vi "Software Commands.vi"() -> ()   [LabVIEW 2015]
panel:
  in  "Aalborg DFC Software Interface Commands":T1(array[cluster])=[{"Command Name"="Mode", "Description"="sets analog mode", "Number"="1", "Command"="M", "Argument 1"="A", "Argument 2"="", "Argument 3"="", "Argument 4"="", "Response"="MA"}, {"Command Name"="Mode", "Description"="set digital mode", "Number"="1", "Command"="M", "Argument 1"="D", "Argument 2"="", "Argument 3"="", "Argument 4"="", "Response"="MD"}, {"Command Name"="Mode", "Description"="returns status", "Number"="1", "Command"="M", "Argument 1"="S", "Argument 2"="", "Argument 3"="", "Argument 4"="", "Response"="MA or MD"}, {"Command Name"="Set Point", "Description"="send desired flow setting (digital mode)", "Number"="2", "Command"="S", "Argument 1"="<Value>", "Argument 2"="", "Argument 3"="", "Argument 4"="", "Response"="S <Value>"}, {"Command Name"="Flow", "Description"="request sensor reading", "Number"="3", "Command"="F", "Argument 1"="", "Argument 2"="", "Argument 3"="", "Argument 4"="", "Response"="<Value>"}, {"Command Name"="Valve", "Description"="R/W op mode of ctl valve - Auto", "Number"="4", "Command"="V", "Argument 1"="A", "Argument 2"="", "Argument 3"="", "Argument 4"="", "Response"="VA"}, {"Command Name"="Valve", "Description"="R/W op mode of ctl valve - Force Open", "Number"="4", "Command"="V", "Argument 1"="O", "Argument 2"="", "Argument 3"="", "Argument 4"="", "Response"="VO"}, {"Command Name"="Valve", "Description"="R/W op mode of ctl valve - Force Closed", "Number"="4", "Command"="V", "Argument 1"="C", "Argument 2"="", "Argument 3"="", "Argument 4"="", "Response"="VC"}, {"Command Name"="Valve", "Description"="R/W op mode of ctl valve - Return Status", "Number"="4", "Command"="V", "Argument 1"="S", "Argument 2"="", "Argument 3"="", "Argument 4"="", "Response"="VA, VO or VC"}, {"Command Name"="Gas Select", "Description"="sel 1/10 gas cals", "Number"="5", "Command"="G", "Argument 1"="<0:1:9>", "Argument 2"="", "Argument 3"="", "Argument 4"="", "Response"="G1 thru G10"}, {"Command Name"="Auto Zero", "Description"="R/W auto zero - enable, do when SP<2%FS", "Number"="6", "Command"="Z", "Argument 1"="E", "Argument 2"="", "Argument 3"="", "Argument 4"="", "Response"="ZE"}, {"Command Name"="Auto Zero", "Description"="R/W auto zero - disable", "Number"="6", "Command"="Z", "Argument 1"="D", "Argument 2"="", "Argument 3"="", "Argument 4"="", "Response"="ZD"}, {"Command Name"="Auto Zero", "Description"="R/W auto zero - do it now", "Number"="6", "Command"="Z", "Argument 1"="N", "Argument 2"="", "Argument 3"="", "Argument 4"="", "Response"="ZN"}, {"Command Name"="Auto Zero", "Description"="R/W auto zero - write zero to SDPROC", "Number"="6", "Command"="Z", "Argument 1"="W", "Argument 2"="", "Argument 3"="", "Argument 4"="", "Response"="ZW"}, {"Command Name"="Auto Zero", "Description"="R/W auto zero - status", "Number"="6", "Command"="Z", "Argument 1"="S", "Argument 2"="", "Argument 3"="", "Argument 4"="", "Response"="ZE, ZD, or ZIN <value>"}, {"Command Name"="Flow Alarms", "Description"="R/W status of gas flow alarms - high dev", "Number"="7", "Command"="A", "Argument 1"="<Value>", "Argument 2"="", "Argument 3"="", "Argument 4"="", "Response"="AH"}, {"Command Name"="Flow Alarms", "Description"="R/W status of gas flow alarms - low dev", "Number"="7", "Command"="A", "Argument 1"="<Value>", "Argument 2"="", "Argument 3"="", "Argument 4"="", "Response"="AL"}, {"Command Name"="Flow Alarms", "Description"="R/W status of gas flow alarms - disable", "Number"="7", "Command"="A", "Argument 1"="", "Argument 2"="", "Argument 3"="", "Argument 4"="", "Response"="AD"}, {"Command Name"="Flow Alarms", "Description"="R/W status of gas flow alarms - status", "Number"="7", "Command"="A", "Argument 1"="", "Argument 2"="", "Argument 3"="", "Argument 4"="", "Response"="N, H, or L"}, {"Command Name"="Relay Action", "Description"="energize relay <Arg 1> when Arg 2 = true - disable", "Number"="8", "Command"="R", "Argument 1"="<1,2>", "Argument 2"="N", "Argument 3"="", "Argument 4"="", "Response"="RN"}, {"Command Name"="Relay Action", "Description"="energize relay <Arg 1> when Arg 2 = true - totalizer > limit", "Number"="8", "Command"="R", "Argument 1"="<1,2>", "Argument 2"="T", "Argument 3"="", "Argument 4"="", "Response"="RT"}, {"Command Name"="Relay Action", "Description"="energize relay <Arg 1> when Arg 2 = true - hi alarm", "Number"="8", "Command"="R", "Argument 1"="<1,2>", "Argument 2"="H", "Argument 3"="", "Argument 4"="", "Response"="RH"}, {"Command Name"="Relay Action", "Description"="energize relay <Arg 1> when Arg 2 = true - lo alarm", "Number"="8", "Command"="R", "Argument 1"="<1,2>", "Argument 2"="L", "Argument 3"="", "Argument 4"="", "Response"="RL"}, {"Command Name"="Relay Action", "Description"="energize relay <Arg 1> when Arg 2 = true - lo < range < hi", "Number"="8", "Command"="R", "Argument 1"="<1,2>", "Argument 2"="R", "Argument 3"="", "Argument 4"="", "Response"="RR"}, {"Command Name"="Relay Action", "Description"="relay <Arg 1> - status", "Number"="8", "Command"="R", "Argument 1"="<1,2>", "Argument 2"="S", "Argument 3"="", "Argument 4"="", "Response"="RN, RT, RH, RL, RR"}, {"Command Name"="Totalizer", "Description"="ctl totalizer - zero", "Number"="9", "Command"="T", "Argument 1"="Z", "Argument 2"="", "Argument 3"="", "Argument 4"="", "Response"="TZ"}, {"Command Name"="Totalizer", "Description"="ctl totalizer - start", "Number"="9", "Command"="T", "Argument 1"="S", "Argument 2"="<N,F>", "Argument 3"="<Value>", "Argument 4"="", "Response"="TSN, TS <value>"}, {"Command Name"="Totalizer", "Description"="ctl totalizer - stop", "Number"="9", "Command"="T", "Argument 1"="P", "Argument 2"="<N,T>", "Argument 3"="<Value>", "Argument 4"="", "Response"="TPN, TPT {N/C} <valve>"}, {"Command Name"="Totalizer", "Description"="ctl totalizer - read", "Number"="9", "Command"="T", "Argument 1"="R", "Argument 2"="", "Argument 3"="", "Argument 4"="", "Response"="<value>"}, {"Command Name"="Totalizer", "Description"="ctl totalizer - disable", "Number"="9", "Command"="T", "Argument 1"="D", "Argument 2"="", "Argument 3"="", "Argument 4"="", "Response"="TD"}, {"Command Name"="K Factors", "Description"="gas correction factor - disable (K = 1)", "Number"="10", "Command"="K", "Argument 1"="D", "Argument 2"="", "Argument 3"="", "Argument 4"="", "Response"="KD"}, {"Command Name"="K Factors", "Description"="gas correction factor - internal table", "Number"="10", "Command"="K", "Argument 1"="I", "Argument 2"="<index>", "Argument 3"="", "Argument 4"="", "Response"="KI <index> <name> <value>"}, {"Command Name"="K Factors", "Description"="gas correction factor - user specified factor", "Number"="10", "Command"="K", "Argument 1"="E", "Argument 2"="<value>", "Argument 3"="", "Argument 4"="", "Response"="KE <value>"}, {"Command Name"="Units", "Description"="set units - %FS", "Number"="11", "Command"="U", "Argument 1"="%", "Argument 2"="", "Argument 3"="", "Argument 4"="", "Response"="U%"}, {"Command Name"="Units", "Description"="set units - SLPM", "Number"="11", "Command"="U", "Argument 1"="SLPM", "Argument 2"="", "Argument 3"="", "Argument 4"="", "Response"="USLPM"}, {"Command Name"="Units", "Description"="set units - SLPH", "Number"="11", "Command"="U", "Argument 1"="SLPH", "Argument 2"="", "Argument 3"="", "Argument 4"="", "Response"="USLPH"}, {"Command Name"="Units", "Description"="set units - MLPM", "Number"="11", "Command"="U", "Argument 1"="MLPM", "Argument 2"="", "Argument 3"="", "Argument 4"="", "Response"="UMLPM"}, {"Command Name"="Units", "Description"="set units - MLPH", "Number"="11", "Command"="U", "Argument 1"="MLPH", "Argument 2"="", "Argument 3"="", "Argument 4"="", "Response"="UMLPH"}, {"Command Name"="Units", "Description"="set units - SCFH", "Number"="11", "Command"="U", "Argument 1"="SCFH", "Argument 2"="", "Argument 3"="", "Argument 4"="", "Response"="USCFH"}, {"Command Name"="Units", "Description"="set units - SCFM", "Number"="11", "Command"="U", "Argument 1"="SCFM", "Argument 2"="", "Argument 3"="", "Argument 4"="", "Response"="USCFM"}, {"Command Name"="Units", "Description"="set units - LBPH", "Number"="11", "Command"="U", "Argument 1"="LBPH", "Argument 2"="", "Argument 3"="", "Argument 4"="", "Response"="ULBPH"}, {"Command Name"="Units", "Description"="set units - LBPM", "Number"="11", "Command"="U", "Argument 1"="LBPM", "Argument 2"="", "Argument 3"="", "Argument 4"="", "Response"="ULBPM"}, {"Command Name"="Units", "Description"="set units - user defined (conversion factor from  SLPM)", "Number"="11", "Command"="U", "Argument 1"="UD", "Argument 2"="<value>", "Argument 3"="<t-base:S,M,H>", "Argument 4"="", "Response"="UUD<value>"}, {"Command Name"="Maintenance Timer", "Description"="Hours since last time unit was calibrated - read", "Number"="12", "Command"="C", "Argument 1"="R", "Argument 2"="", "Argument 3"="", "Argument 4"="", "Response"="<value>"}, {"Command Name"="Maintenance Timer", "Description"="Hours since last time unit was calibrated - reset", "Number"="12", "Command"="C", "Argument 1"="C", "Argument 2"="", "Argument 3"="", "Argument 4"="", "Response"="CC"}, {"Command Name"="Full Scale", "Description"="return FS-rated flow in SLPM", "Number"="13", "Command"="E", "Argument 1"="", "Argument 2"="", "Argument 3"="", "Argument 4"="", "Response"="<value>"}, {"Command Name"="Read Memory", "Description"="read value in memory", "Number"="14", "Command"="MR", "Argument 1"="<index:0:999>", "Argument 2"="", "Argument 3"="", "Argument 4"="", "Response"="<value>"}, {"Command Name"="Write Memory", "Description"="write value to memory", "Number"="15", "Command"="MW", "Argument 1"="<index:0:999>", "Argument 2"="<value>", "Argument 3"="", "Argument 4"="", "Response"="MMXXX<value> XXX=index"}, {"Command Name"="Auto Tune", "Description"="performs Auto Tune", "Number"="16", "Command"="AT", "Argument 1"="<Value>", "Argument 2"="", "Argument 3"="", "Argument 4"="", "Response"="AT<value>"}, {"Command Name"="Auto Tune", "Description"="read Auto Tune status", "Number"="16", "Command"="S", "Argument 1"="", "Argument 2"="", "Argument 3"="", "Argument 4"="", "Response"="ATSI <Kp,Ki,Kd> (in progress); ATSD <Kp,Ki,Kd> (done)"}]
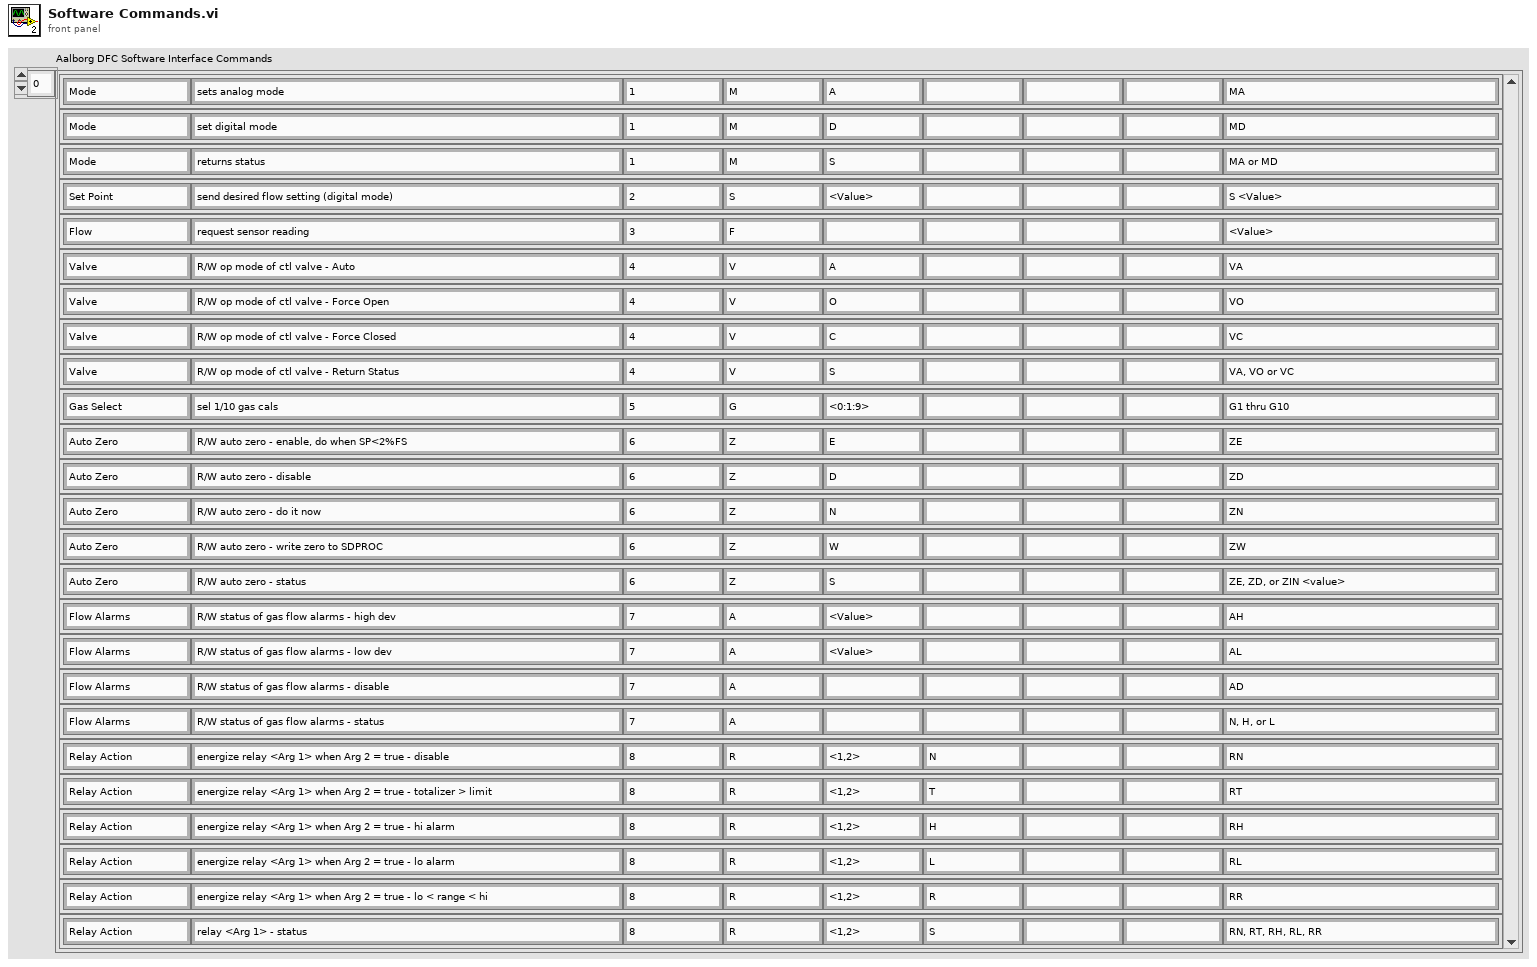
[diagram p1: front panel]
types:
  T1 = cluster{"Command Name":string, "Description":string, "Number":string, "Command":string, "Argument 1":string, "Argument 2":string, "Argument 3":string, "Argument 4":string, "Response":string}[]
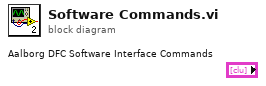
[diagram p0: block diagram]
diagram:
